vi "IPS120 WH2 - Write Setpoint.vi"(0 "Setpoint":dbl format="%.3f", 1 "GPIB Address":string) -> ()   [LabVIEW 2009]
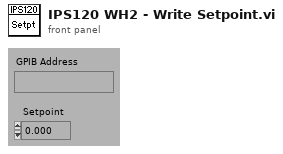
[diagram p1: front panel]
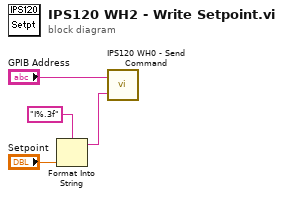
[diagram p0: block diagram]
diagram:
  n1 = Format Into String(format string="I%.3f", "Setpoint") -> (resulting string=w1:string)  [unwired: 2 in, 1 out]
  n2 = call "IPS120 WH0 - Send Command.vi"("Command String"=w1, "GPIB Address"="GPIB Address") -> ()  [unwired: 1 out]
